vi "Add TX Packet to Stats.vi"(7 "Packet":string, 8 "error in (no error)":errorcluster, 11 "Name":string) -> (0 "error out":errorcluster)   [LabVIEW 2023, in "WebSocket.lvclass"]
uses:
  WebSocket.lvclass
  WebSocket Stats VIG Mode.ctl
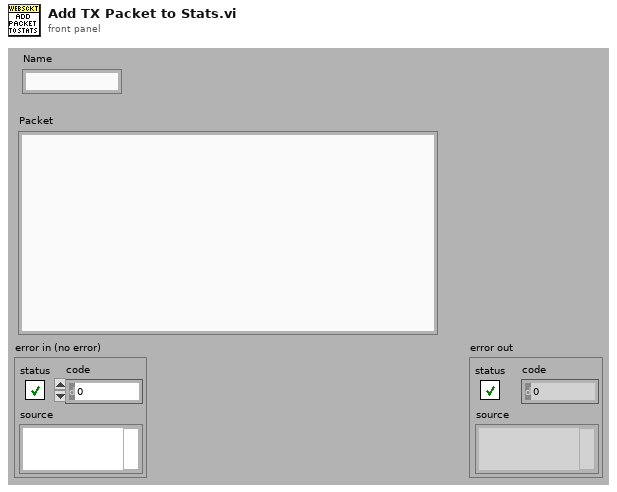
[diagram p1: front panel]
types:
  T1 = typedef "WebSocket Stats VIG Mode.ctl" = enum16{"Init", "Set", "Update", "Get All"}
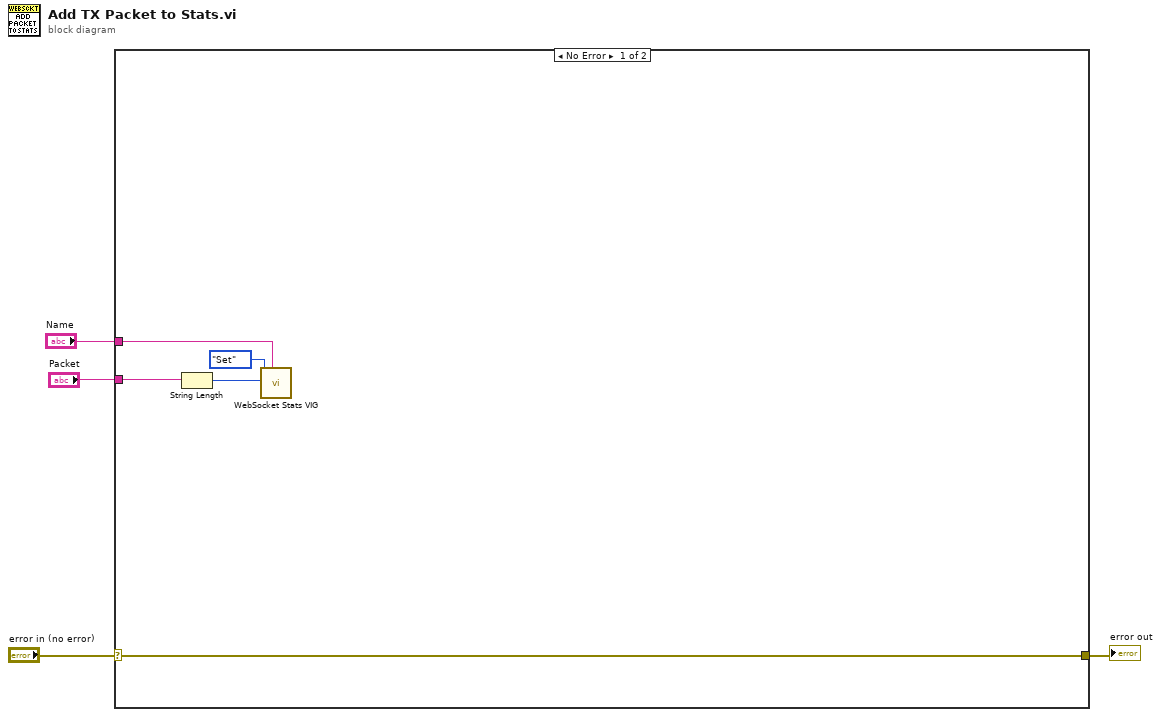
[diagram p0: block diagram]
diagram:
  n1 = case shown="No Error" "error in (no error)" {
    selector: "error in (no error)" -> [w8 w10]
    tunnel: [w8 w10] -> w3
    tunnel: "Packet" -> [w9 _]
    tunnel: "Name" -> [w6 _]
    frame No Error {
      n2 = String Length(string=w9) -> (length=w7:i32)
      n3 = call "WebSocket Stats VIG.vi"("Name"=w6, "Length"=w7, "mode"=WebSocket_Stats_VIG_Mode."Set") -> ()  [unwired: 6 in, 3 out]
    }
    frame Error {
    }
  }
  "error out" <- w3
